vi "appendToExisting.vi"(8 "error in (no error)":errorcluster, 11 "xwpfDocument in":refnum<class "xwpfDocument.lvclass">) -> (0 "error out":errorcluster, 3 "xwpfDocument out":refnum<class "xwpfDocument.lvclass">)   [LabVIEW 2017, in "Word_Specific.lvlib" / "xwpfDocument.lvclass"]
uses:
  xwpfDocument.lvclass
  xwpfDocument.lvclass/xwpfDocument.ctl
  C:/Users/Neo/Desktop/Dev_Tools_BR/LabVIEW_NPOI/lib/NPOI 2.1.1/NPOI.OOXML.dll
  lib/NPOI 2.1.1/NPOI.OOXML.dll
  xwpfParagraph/xwpfParagraph.lvclass
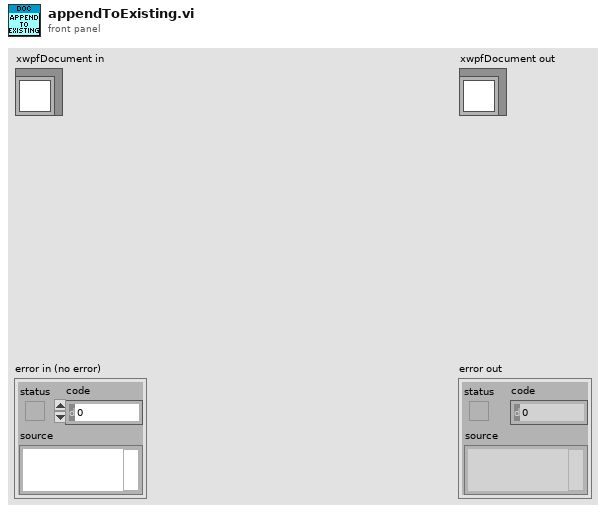
[diagram p1: front panel]
types:
  T1 = enum16{"Title", "Heading 1", "Heading 2", "Heading 3", "Normal", "Figure", "Page Break"}
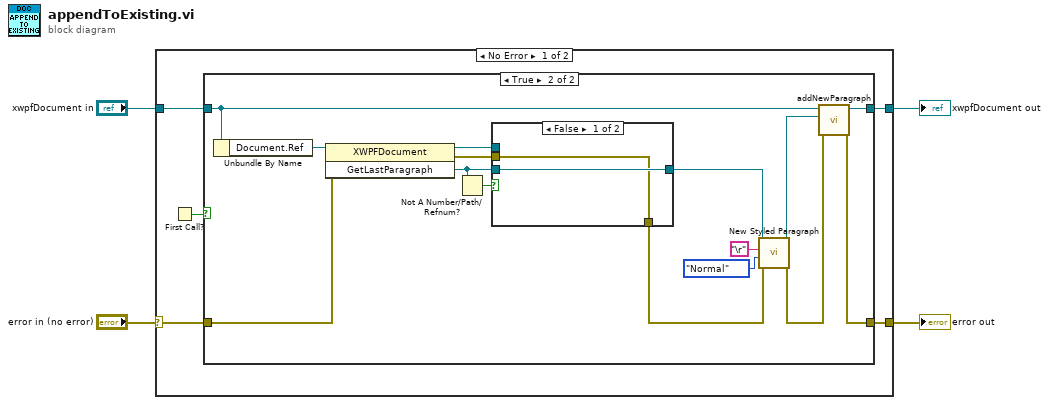
[diagram p0: block diagram]
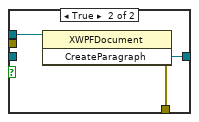
[diagram p3: hidden frame]
diagram:
  n1 = case shown="No Error" "error in (no error)" {
    selector: "error in (no error)" -> [w7 w33]
    tunnel: [w6 w33] -> w3
    tunnel: [w8 w32] -> w1
    tunnel: "xwpfDocument in" -> [w9 w32]
    frame No Error {
      n2 = First Call?() -> (First Call?: T/F=w5:bool)
      n3 = case shown="True" w5 {
        tunnel: w9 -> [w11 w21]
        tunnel: [w11 w20] -> w8
        tunnel: w7 -> [w10 w17]
        tunnel: [w10 w14] -> w6
        frame False {
        }
        frame True {
          n4 = Unbundle By Name(w21) -> ("Document.Ref"=w23:refnum<k24>)
          n5 = invoke class="XWPFDocument" method="GetLastParagraph"(reference=w23, error in=w17) -> (reference out=w26:refnum<k24>, error out=w24:errorcluster, "GetLastParagraph"=w25:refnum<k24>)  [unwired: 1 in]
          n6 = Not A Number/Path/Refnum?(number/path/refnum=w25) -> (NaN/Path/Refnum?=w22:bool)
          n7 = case shown="False" w22 {
            tunnel: w26 -> [_ w31]
            tunnel: [w28 w30] -> w19
            tunnel: w25 -> [w28 _]
            tunnel: w24 -> [w27 _]
            tunnel: [w27 w29] -> w16
            frame False {
            }
            frame True {
              n8 = invoke class="XWPFDocument" method="CreateParagraph"(reference=w31) -> (error out=w29:errorcluster, "CreateParagraph"=w30:refnum<k24>)  [unwired: 2 in, 1 out]
            }
          }
          n9 = call "New Styled Paragraph.vi"("error in (no error)"=w16, "Type"=T1."Normal", "Paragraph.Text"="\r", "Paragraph.Ref"=w19) -> ("error out"=w15:errorcluster, "xwpfParagraph out"=w18:refnum<class "xwpfParagraph.lvclass">)  [unwired: 6 in]
          n10 = call "addNewParagraph.vi"("error in (no error)"=w15, "New Paragraph"=w18, "xwpfDocument in"=w21) -> ("error out"=w14:errorcluster, "xwpfDocument out"=w20:refnum<class "xwpfDocument.lvclass">)  [unwired: 7 in]
        }
      }
    }
    frame Error {
    }
  }
  "error out" <- w3
  "xwpfDocument out" <- w1
